vi "Diff_Drive_System_Act_AutoTune.vi"(6 "FPGA_Time_Seconds":dbl, 9 "Right Speed":dbl, 10 "Left Speed":dbl, 11 "Diff_Drive_Device_Refs":T1 {"GyroDevRef"."Sample Rate" min=0.25 max=100.0 step=0.25}) -> ()   [LabVIEW 2019]
uses:
  Diff_Drive_System_Device_Refs.ctl
  <vilib>/Rock Robotics/WPI/Gyro/WPI_GyroDevRef.ctl
  <vilib>/Rock Robotics/SystemInterfaces/AI/FPGA_AIChannel.ctl
  <vilib>/Rock Robotics/SystemInterfaces/spilib/spi_bus.ctl
  <vilib>/Rock Robotics/WPI/RobotDrive/WPI_RobotDriveDevRef.ctl
  <vilib>/Rock Robotics/WPI/MotorControl/WPI_MotorControlDeviceRef.ctl
  <vilib>/Rock Robotics/WPI/MotorControl/WPI_MotorControlType.ctl
  <vilib>/Rock Robotics/SystemInterfaces/DIO/FPGA_DIOPWMChannel.ctl
  <vilib>/Rock Robotics/WPI/PWM/WPI_PWMDeadband.ctl
  <vilib>/Rock Robotics/SystemInterfaces/DIO/FPGA_DIOChannel.ctl
  <vilib>/Rock Robotics/WPI/Encoder/WPI_EncoderDevRef.ctl
  <vilib>/Rock Robotics/SystemInterfaces/Encoder/FPGA_EncoderIdx.ctl
  <vilib>/Rock Robotics/SystemInterfaces/Counter/FPGA_CounterCtrSystemIndex.ctl
  <vilib>/Rock Robotics/WPI/Encoder/WPI_EncoderType.ctl
  <vilib>/Rock Robotics/WPI/ThirdParty/JAS_Junk/TrajLib/SlewRateLimiter_New.vi
  <vilib>/Rock Robotics/WPI/ThirdParty/JAS_Junk/TrajLib/SlewRateLimiter_Reset.vi
  <vilib>/Rock Robotics/WPI/ThirdParty/JAS_Junk/TrajLib/SlewRateLimiter_Calculate.vi
  <vilib>/Rock Robotics/WPI/ThirdParty/JAS_Junk/TrajLib/SlewRateLimiter_SetRate.vi
  <vilib>/Rock Robotics/WPI/ThirdParty/JAS_Junk/TrajLib/SimpleMotorFF_Calculate.vi
  <vilib>/Rock Robotics/WPI/ThirdParty/JAS_Junk/TrajLib/PIDController_AtSetpoint.vi
  <vilib>/Rock Robotics/WPI/ThirdParty/JAS_Junk/TrajLib/PIDController_SetPIDF.vi
  <vilib>/Rock Robotics/WPI/ThirdParty/JAS_Junk/TrajLib/PIDController_SetDerivativeFilter.vi
  <vilib>/Rock Robotics/WPI/ThirdParty/JAS_Junk/TrajLib/PIDController_SetIntegratorRange.vi
  <vilib>/Rock Robotics/WPI/ThirdParty/JAS_Junk/TrajLib/PIDController_SetTolerancePandV.vi
  <vilib>/Rock Robotics/WPI/ThirdParty/JAS_Junk/TrajLib/PIDController_DisableContinousInput.vi
  <vilib>/Rock Robotics/WPI/ThirdParty/JAS_Junk/TrajLib/PIDController_EnableContinousInput.vi
  <vilib>/Rock Robotics/WPI/ThirdParty/JAS_Junk/TrajLib/PIDController_Reset.vi
  <vilib>/Rock Robotics/WPI/ThirdParty/JAS_Junk/TrajLib/PIDController_New.vi
  <vilib>/Rock Robotics/WPI/ThirdParty/JAS_Junk/TrajLib/PIDController_SetOutputLimits.vi
  <vilib>/Rock Robotics/WPI/ThirdParty/JAS_Junk/TrajLib/PIDController_NewPeriod.vi
  <vilib>/Rock Robotics/SystemInterfaces/NetworkCommunication/NetComm_UsageReport_report.vi
  Diff_Drive_System_Globals.vi
  <vilib>/Rock Robotics/WPI/ThirdParty/JAS_Junk/TrajLib/Util_LibraryGlobals.vi
  <vilib>/Rock Robotics/WPI/ThirdParty/JAS_Junk/TrajLib/PIDController_AdvCalculate_FF_Sp_Pv.vi
  <vilib>/Rock Robotics/WPI/ThirdParty/JAS_Junk/TrajLib/Trajectory_Library.lvlib
panel:
  # "Analog"
  # "XRS"
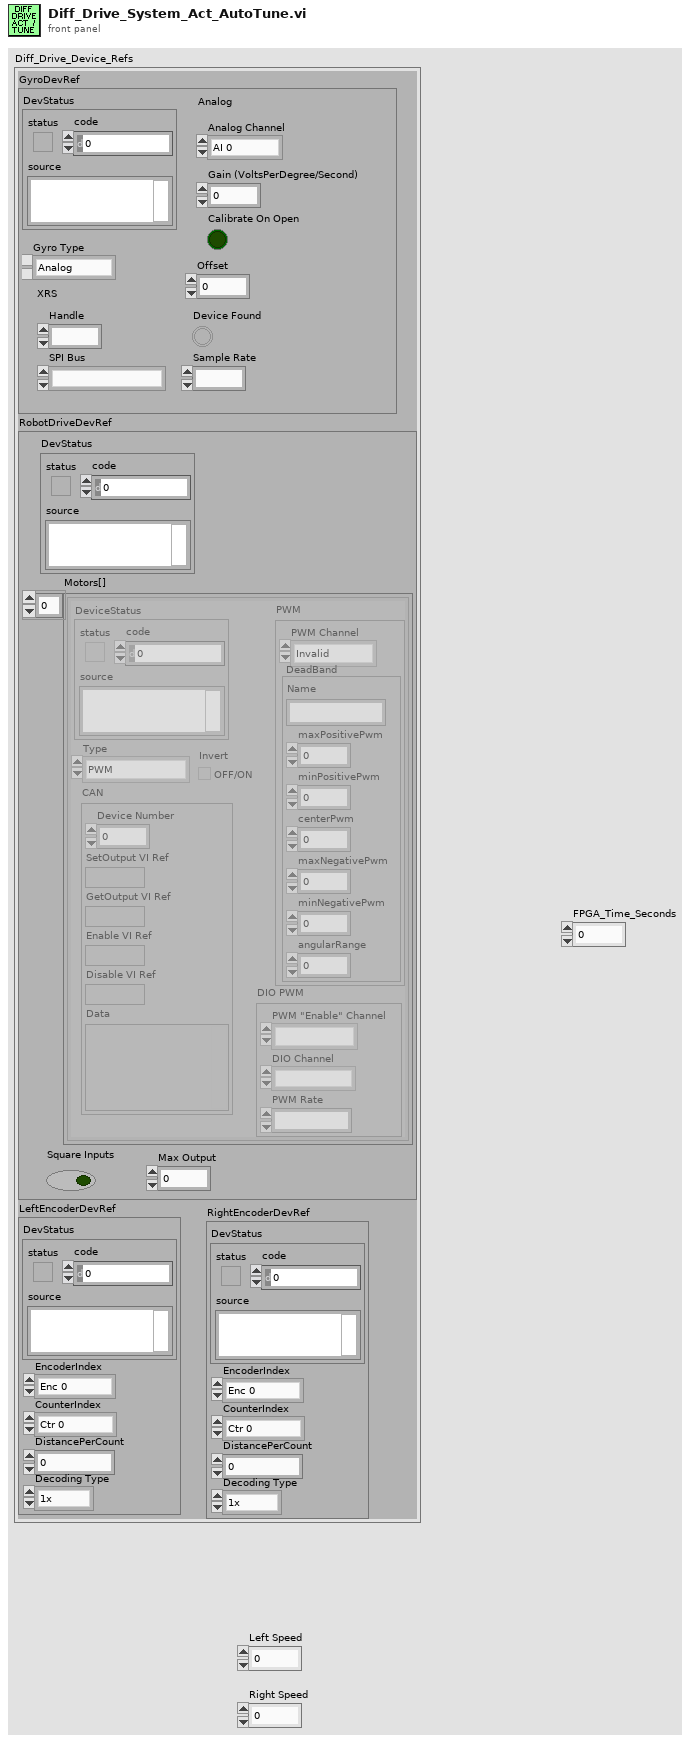
[diagram p1: front panel]
types:
  T1 = typedef "Diff_Drive_System_Device_Refs.ctl" = cluster{"GyroDevRef":T2, "RobotDriveDevRef":T5, "LeftEncoderDevRef":T11, "RightEncoderDevRef":T11}
  T2 = typedef "WPI_GyroDevRef.ctl" = cluster{"DevStatus":errorcluster, "Analog Channel":T3, "Gain (VoltsPerDegree/Second)":dbl, "Gyro Type":enum16{"Analog", "XRS450"}, "Handle":i32, "SPI Bus":T4, "Device Found":bool, "Sample Rate":dbl, "Calibrate On Open":bool, "Offset":dbl}
  T3 = typedef "FPGA_AIChannel.ctl" = enum8{"AI 0", "AI 1", "AI 2", "AI 3", "AI MXP 0", "AI MXP 1", "AI MXP 2", "AI MXP 3", "Invalid"}
  T4 = typedef "spi_bus.ctl" = enum16{"SPI On-Board, CS0", "SPI On-Board, CS1", "SPI On-Board, CS2", "SPI On-Board, CS3", "SPI MXP", "Invalid"}
  T5 = typedef "WPI_RobotDriveDevRef.ctl" = cluster{"DevStatus":errorcluster, "Motors[]":T6[], "Square Inputs":bool, "Max Output":dbl}
  T6 = typedef "WPI_MotorControlDeviceRef.ctl" = cluster{"DeviceStatus":errorcluster, "Type":T7, "PWM":cluster{"PWM Channel":T8, "DeadBand":T9}, "CAN":cluster{"Device Number":u8, "SetOutput VI Ref":variant, "GetOutput VI Ref":variant, "Enable VI Ref":variant, "Disable VI Ref":variant, "Data":variant}, "Invert":bool, "DIO PWM":cluster{"PWM \"Enable\" Channel":T8, "DIOChannel":T10, "PWM Rate":dbl}}
  T7 = typedef "WPI_MotorControlType.ctl" = enum16{"PWM", "CAN", "DIO PWM"}
  T8 = typedef "FPGA_DIOPWMChannel.ctl" = enum8{"PWM 0", "PWM 1", "PWM 2", "PWM 3", "PWM 4", "PWM 5", "PWM 6", "PWM 7", "PWM 8", "PWM 9", "PWM MXP 0", "PWM MXP 1", "PWM MXP 2", "PWM MXP 3", "PWM MXP 4", "PWM MXP 5", "PWM MXP 6", "PWM MXP 7", "PWM MXP 8", "PWM MXP 9", "Invalid"}
  T9 = typedef "WPI_PWMDeadband.ctl" = cluster{"Name":string, "maxPositivePwm":i32, "minPositivePwm":i32, "centerPwm":i32, "maxNegativePwm":i32, "minNegativePwm":i32, "angularRange":u16}
  T10 = typedef "FPGA_DIOChannel.ctl" = enum8{"DIO 0", "DIO 1", "DIO 2", "DIO 3", "DIO 4", "DIO 5", "DIO 6", "DIO 7", "DIO 8", "DIO 9", "DIO MXP 0", "DIO MXP 1", "DIO MXP 2", "DIO MXP 3", "DIO MXP 4", "DIO MXP 5", "DIO MXP 6", "DIO MXP 7", "DIO MXP 8", "DIO MXP 9", "DIO MXP 10", "DIO MXP 11", "DIO MXP 12", "DIO MXP 13", "DIO MXP 14", "DIO MXP 15", "SPI Port CS1", "SPI Port CS2", "SPI Port CS3", "SPI Port MISO", "SPI Port MOSI", "Invalid"}
  T11 = typedef "WPI_EncoderDevRef.ctl" = cluster{"DevStatus":errorcluster, "EncoderIndex":T12, "CounterIndex":T13, "DistancePerCount":dbl, "Decoding Type":T14}
  T12 = typedef "FPGA_EncoderIdx.ctl" = enum8{"Enc 0", "Enc 1", "Enc 2", "Enc 3", "Enc 4", "Enc 5", "Enc 6", "Enc 7", "Invalid"}
  T13 = typedef "FPGA_CounterCtrSystemIndex.ctl" = enum8{"Ctr 0", "Ctr 1", "Ctr 2", "Ctr 3", "Ctr 4", "Ctr 5", "Ctr 6", "Ctr 7", "Invalid"}
  T14 = typedef "WPI_EncoderType.ctl" = enum16{"1x", "2x", "4x"}
  T15 = enum16{"Ziegler Nicols - Fast", "Ziegler Nicols - Normal", "Ziegler Nicols - Slow", "CHR regulator - 0% overshoot", "CHR regulator - 20% overshoot", "CHR servo - 0 % overshoot", "CHR servo - 20% overshoot"}
  T16 = typedef "Trajectory_Library.lvlib/SIMPLE_MOTOR_FF.ctl" = cluster{"Ks":dbl, "Kv":dbl, "Ka":dbl, "KnInv":dbl}
  T17 = typedef "Trajectory_Library.lvlib/PID_ADV_LIMITS.ctl" = cluster{"MaxInput":dbl, "MinInput":dbl, "Continuous":bool, "MaxOutput":dbl, "MinOutput":dbl}
  T18 = typedef "Trajectory_Library.lvlib/PID_ADV_TUNING.ctl" = cluster{"Kf":dbl, "Kp":dbl, "Ki":dbl, "Kd":dbl, "MaximumIntegral":dbl, "MinimumIntegral":dbl, "Filter Derivative":bool}
  T19 = cluster{"Controller Constant Type":enum16{"Ziegler Nicols - Fast", "Ziegler Nicols - Normal", "Ziegler Nicols - Slow", "CHR regulator - 0% overshoot", "CHR regulator - 20% overshoot", "CHR servo - 0 % overshoot", "CHR servo - 20% overshoot"}, "Type of Controller":enum16{"P", "PI", "PID"}, "CO Offset":dbl, "Kn":dbl, "Tuning Tolerance":dbl, "Plant Tolerance":dbl, "Newest Avg Time ":i32, "Long Ave Time":i32}
  T20 = cluster{"proportional gain (Kp)":dbl, "integral time (Ki / Sec)":dbl, "derivative time (Kd /Sec)":dbl}
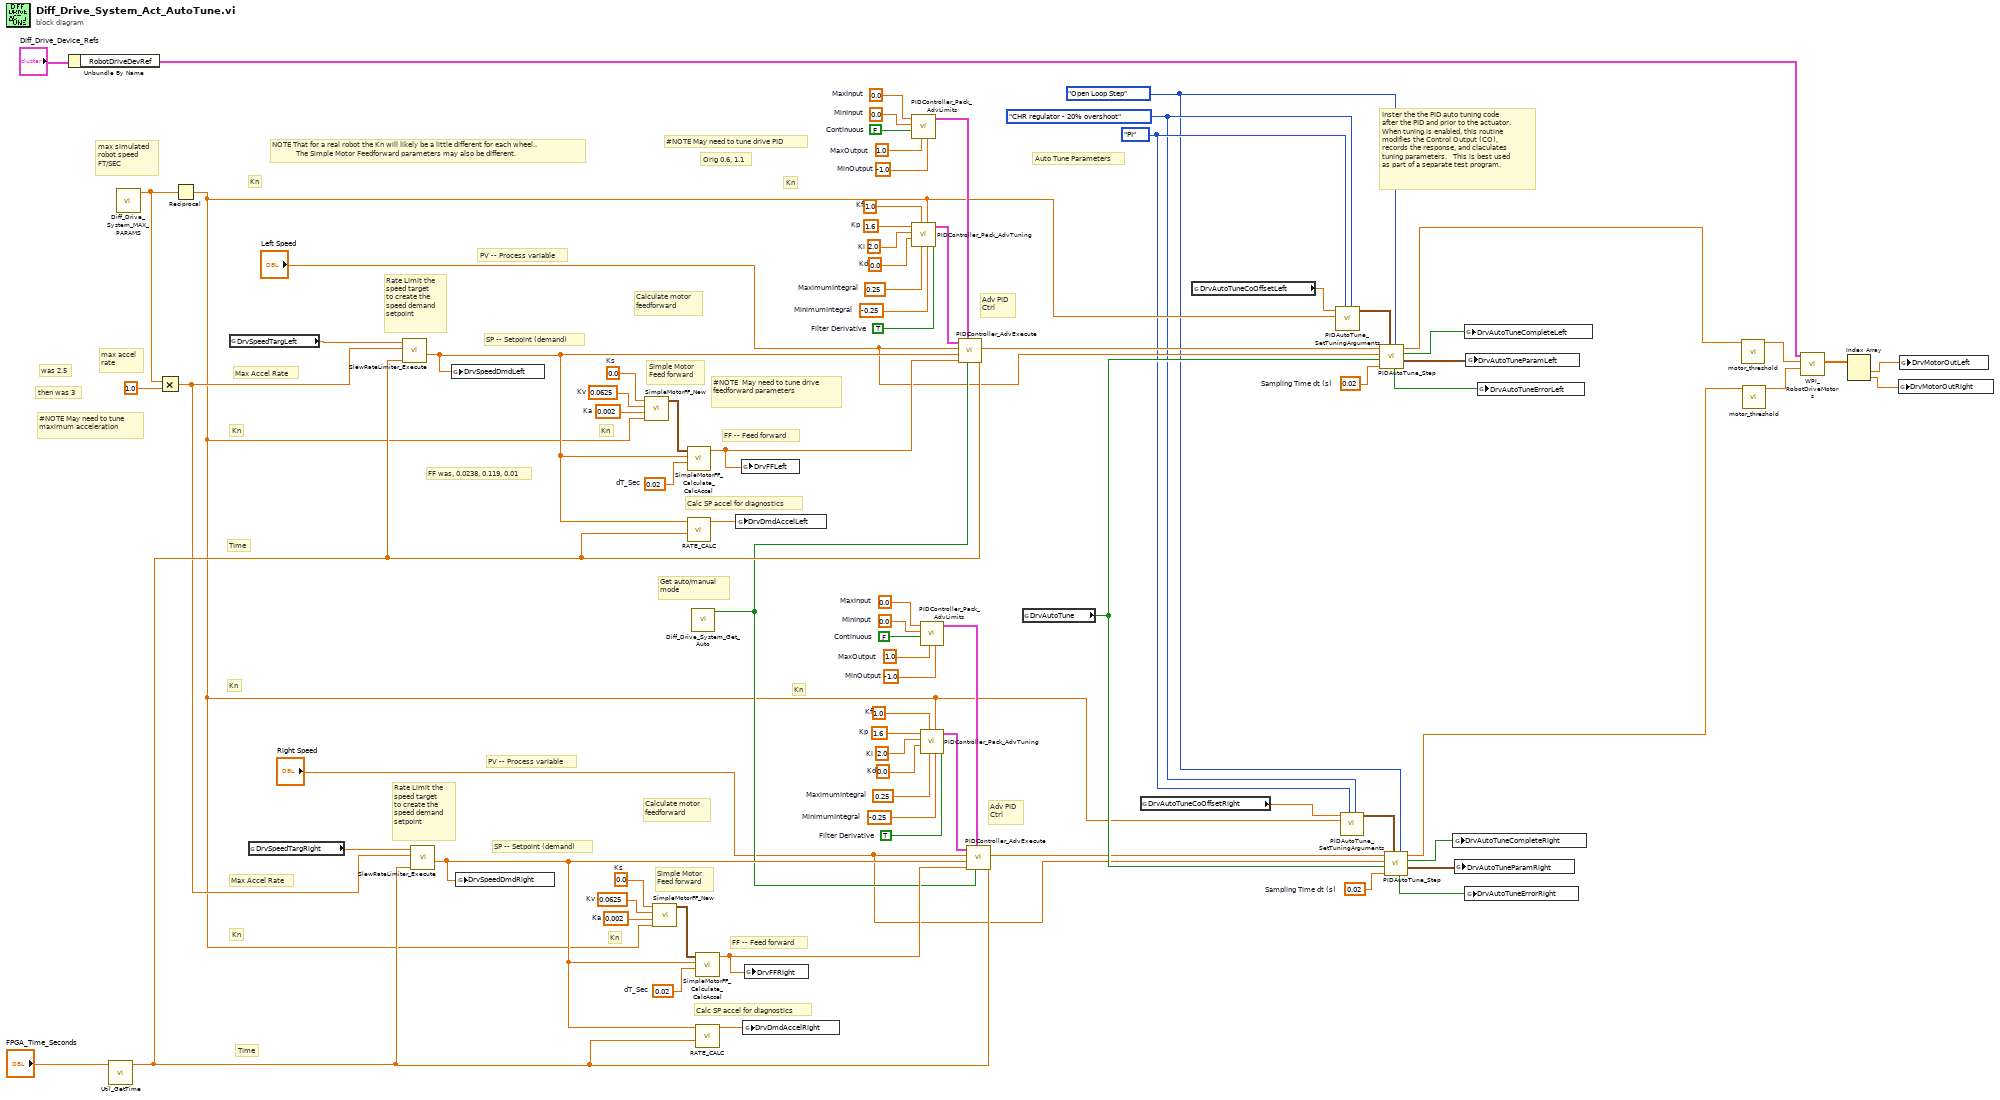
[diagram p0: block diagram]
diagram:
  w19 = 0.02  # Sampling Time dt (s)
  w1 = enum16{"Open Loop Step", "Closed Loop Step"}."Open Loop Step" ("Procedure Type")
  w2 = T15."CHR regulator - 20% overshoot" ("Controller Constant Type")
  w3 = enum16{"P", "PI", "PID"}."PI" ("Type of Controller")
  w24 = 0.02  # Sampling Time dt (s)
  w45 = 1.6  # Kp
  w44 = 2.0  # Ki
  w43 = 0.0  # Kd
  w42 = 1.0  # Kf
  w41 = 0.25  # MaximumIntegral
  w40 = -0.25  # MinimumIntegral
  w39 = TRUE  # Filter Derivative
  w37 = 0.0  # MinInput
  w36 = FALSE  # Continuous
  w35 = 1.0  # MaxOutput
  w38 = -1.0  # MinOutput
  w34 = 0.0  # MaxInput
  w50 = 0.02  # dT_Sec
  w48 = 0.0  # Ks
  w47 = 0.0625  # Kv
  w46 = 0.002  # Ka
  w68 = 1.6  # Kp
  w67 = 2.0  # Ki
  w66 = 0.0  # Kd
  w65 = 1.0  # Kf
  w64 = 0.25  # MaximumIntegral
  w63 = -0.25  # MinimumIntegral
  w62 = TRUE  # Filter Derivative
  w60 = 0.0  # MinInput
  w59 = FALSE  # Continuous
  w58 = 1.0  # MaxOutput
  w61 = -1.0  # MinOutput
  w57 = 0.0  # MaxInput
  w74 = 0.02  # dT_Sec
  w72 = 0.0  # Ks
  w71 = 0.0625  # Kv
  w70 = 0.002  # Ka
  # "Auto Tune Parameters"
  # "Inster the the PID auto tuning code\nafter the PID and prior to the actuator.\nWhen tuning is enabled, this routine\nmodifies the Control Output (CO), \nrecords the response, and claculates\ntuning parameters.   This is best used\nas part of a separate test program."
  # "Get auto/manual\nmode"
  # "then was 3"
  # "FF was, 0.0238, 0.119, 0.01"
  # "Orig 0.6, 1.1"
  # "NOTE That for a real robot the Kn will likely be a little different for each wheel..\n            The Simple Motor Feedforward parameters may also be different."
  # "Max Accel Rate"
  # "Max Accel Rate"
  # "Time"
  # "Kn"
  # "Kn"
  # "Kn"
  # "Kn"
  # "Time"
  # "Kn"
  # "PV -- Process variable"
  # "Kn"
  # "Calc SP accel for diagnostics"
  # "FF -- Feed forward"
  # "SP -- Setpoint (demand)"
  # "Adv PID\nCtrl"
  # "Calculate motor\nfeedforward"
  # "Rate Limit the \nspeed target\nto create the\nspeed demand\nsetpoint"
  # "Simple Motor\nFeed forward"
  # "Kn"
  # "PV -- Process variable"
  # "Kn"
  # "Calc SP accel for diagnostics"
  # "FF -- Feed forward"
  # "SP -- Setpoint (demand)"
  # "Adv PID\nCtrl"
  # "Calculate motor\nfeedforward"
  # "was 2.5"
  # "Rate Limit the \nspeed target\nto create the\nspeed demand\nsetpoint"
  # "Simple Motor\nFeed forward"
  # "#NOTE May need to tune drive PID"
  # "#NOTE May need to tune maximum acceleration"
  # "#NOTE  May need to tune drive feedforward parameters"
  # "max simulated\nrobot speed\nFT/SEC"
  # "max accel\nrate"
  n1 = Unbundle By Name("Diff_Drive_Device_Refs") -> ("RobotDriveDevRef"=w77:T5)
  n2 = call <vilib>:"Util_GetTime.vi"("Pass_Through_Time"="FPGA_Time_Seconds") -> ("FPGA_Time_Seconds"=w31:dbl)  [unwired: 9 in, 1 out]
  n3 = call "Diff_Drive_System_MAX_PARAMS.vi"() -> ("Max Speed Ft/Sec"=w52:dbl)  [unwired: 9 in, 2 out]
  n4 = Multiply(x=w52, y=1.0 ("x")) -> (x*y=w30:dbl)
  n5 = Reciprocal(x=w52) -> (1/x=w12:dbl)
  n6 = global read "Diff_Drive_System_Globals.vi" "DrvSpeedTargLeft"() -> (w69:dbl)
  n7 = global read "Diff_Drive_System_Globals.vi" "DrvSpeedTargRight"() -> (w29:dbl)
  n8 = call <vilib>:"SlewRateLimiter_Execute.vi"("Time"=w31, "PositiveRate"=w30, "Input"=w69) -> ("Output"=w54:dbl)  [unwired: 7 in, 1 out]
  n9 = call <vilib>:"SlewRateLimiter_Execute.vi"("Time"=w31, "PositiveRate"=w30, "Input"=w29) -> ("Output"=w26:dbl)  [unwired: 7 in, 1 out]
  n10 = global write "Diff_Drive_System_Globals.vi" "DrvSpeedDmdLeft"(w54) -> ()
  n11 = global write "Diff_Drive_System_Globals.vi" "DrvSpeedDmdRight"(w26) -> ()
  n12 = call <vilib>:"SimpleMotorFF_New.vi"("Kn"=w12, "Ka"=w70, "Kv"=w71, "Ks"=w72) -> ("SIMPLE_MOTOR_FF"=w73:T16)  [unwired: 7 in]
  n13 = call <vilib>:"SimpleMotorFF_New.vi"("Kn"=w12, "Ka"=w46, "Kv"=w47, "Ks"=w48) -> ("SIMPLE_MOTOR_FF"=w49:T16)  [unwired: 7 in]
  n14 = call <vilib>:"SimpleMotorFF_Calculate_CalcAccel.vi"("dT_Sec"=w74, "VelSp"=w54, "SIMPLE_MOTOR_FF"=w73) -> ("FeedForward"=w51:dbl)  [unwired: 8 in]
  n15 = call "RATE_CALC.vi"("Time"=w31, "Input"=w54) -> ("Output"=w53:dbl)  [unwired: 9 in]
  n16 = call "Diff_Drive_System_Get_Auto.vi"() -> ("Auto Mode"=w25:bool)  [unwired: 11 in]
  n17 = call <vilib>:"SimpleMotorFF_Calculate_CalcAccel.vi"("dT_Sec"=w50, "VelSp"=w26, "SIMPLE_MOTOR_FF"=w49) -> ("FeedForward"=w28:dbl)  [unwired: 8 in]
  n18 = call "RATE_CALC.vi"("Time"=w31, "Input"=w26) -> ("Output"=w27:dbl)  [unwired: 9 in]
  n19 = global write "Diff_Drive_System_Globals.vi" "DrvDmdAccelLeft"(w53) -> ()
  n20 = global write "Diff_Drive_System_Globals.vi" "DrvFFLeft"(w51) -> ()
  n21 = global write "Diff_Drive_System_Globals.vi" "DrvDmdAccelRight"(w27) -> ()
  n22 = global write "Diff_Drive_System_Globals.vi" "DrvFFRight"(w28) -> ()
  n23 = call <vilib>:"PIDController_Pack_AdvLimits.vi"("MinOutput"=w61, "MaxOutput"=w58, "Continuous"=w59, "MinInput"=w60, "MaxInput"=w57) -> ("Adv PID Limits"=w55:T17)  [unwired: 6 in]
  n24 = call <vilib>:"PIDController_Pack_AdvTuning.vi"("Filter Derivative"=w62, "MinimumIntegral"=w63, "Kn"=w12, "MaximumIntegral"=w64, "Kf"=w65, "Kd"=w66, "Ki"=w67, "Kp"=w68) -> ("Adv PID Tuning"=w56:T18)  [unwired: 3 in]
  n25 = call <vilib>:"PIDController_Pack_AdvLimits.vi"("MinOutput"=w38, "MaxOutput"=w35, "Continuous"=w36, "MinInput"=w37, "MaxInput"=w34) -> ("Adv PID Limits"=w32:T17)  [unwired: 6 in]
  n26 = call <vilib>:"PIDController_Pack_AdvTuning.vi"("Filter Derivative"=w39, "MinimumIntegral"=w40, "Kn"=w12, "MaximumIntegral"=w41, "Kf"=w42, "Kd"=w43, "Ki"=w44, "Kp"=w45) -> ("Adv PID Tuning"=w33:T18)  [unwired: 3 in]
  n27 = call <vilib>:"PIDController_AdvExecute.vi"("Time"=w31, "Auto"=w25, "Adv PID Limits"=w55, "FF-FeedForward"=w51, "SP-SetPoint"=w54, "PV-Measurement"="Left Speed", "Adv PID Tuning"=w56) -> ("CO-ControlOutput"=w21:dbl)  [unwired: 2 in, 2 out]
  n28 = call <vilib>:"PIDController_AdvExecute.vi"("Time"=w31, "Auto"=w25, "Adv PID Limits"=w32, "FF-FeedForward"=w28, "SP-SetPoint"=w26, "PV-Measurement"="Right Speed", "Adv PID Tuning"=w33) -> ("CO-ControlOutput"=w16:dbl)  [unwired: 2 in, 2 out]
  n29 = global read "Diff_Drive_System_Globals.vi" "DrvAutoTune"() -> (w17:bool)
  n30 = global read "Diff_Drive_System_Globals.vi" "DrvAutoTuneCoOffsetRight"() -> (w13:dbl)
  n31 = global read "Diff_Drive_System_Globals.vi" "DrvAutoTuneCoOffsetLeft"() -> (w14:dbl)
  n32 = call <vilib>:"PIDAutoTune_SetTuningArguments.vi"("Controller Constant Type"=w2, "Type of Controller"=w3, "Kn"=w12, "CO Offset"=w14) -> ("Configuration Parameters"=w23:T19)  [unwired: 7 in]
  n33 = call <vilib>:"PIDAutoTune_SetTuningArguments.vi"("Controller Constant Type"=w2, "Type of Controller"=w3, "Kn"=w12, "CO Offset"=w13) -> ("Configuration Parameters"=w18:T19)  [unwired: 7 in]
  n34 = call <vilib>:"PIDAutoTune_Step.vi"("Procedure Type"=w1, "Configuration Parameters"=w23, "Sampling Time dt (s)"=w24, "Tune"=w17, "Measurement  (PV)"="Left Speed", "Control Output (Co)"=w21) -> ("New Tuning Parameters"=w10:T20, "Tuning Done"=w11:bool, "Adj CO"=w20:dbl, "Error Occured"=w4:bool)  [unwired: 2 out]
  n35 = call <vilib>:"PIDAutoTune_Step.vi"("Procedure Type"=w1, "Configuration Parameters"=w18, "Sampling Time dt (s)"=w19, "Tune"=w17, "Measurement  (PV)"="Right Speed", "Control Output (Co)"=w16) -> ("New Tuning Parameters"=w8:T20, "Tuning Done"=w9:bool, "Adj CO"=w15:dbl, "Error Occured"=w5:bool)  [unwired: 2 out]
  n36 = global write "Diff_Drive_System_Globals.vi" "DrvAutoTuneCompleteRight"(w9) -> ()
  n37 = global write "Diff_Drive_System_Globals.vi" "DrvAutoTuneParamRight"(w8) -> ()
  n38 = global write "Diff_Drive_System_Globals.vi" "DrvAutoTuneCompleteLeft"(w11) -> ()
  n39 = global write "Diff_Drive_System_Globals.vi" "DrvAutoTuneErrorRight"(w5) -> ()
  n40 = global write "Diff_Drive_System_Globals.vi" "DrvAutoTuneParamLeft"(w10) -> ()
  n41 = global write "Diff_Drive_System_Globals.vi" "DrvAutoTuneErrorLeft"(w4) -> ()
  n42 = call "motor_threshold.vi"("motor in"=w20) -> ("motor out"=w22:dbl)  [unwired: 10 in]
  n43 = call "motor_threshold.vi"("motor in"=w15) -> ("motor out"=w81:dbl)  [unwired: 10 in]
  n44 = call <vilib>:"WPI_RobotDriveMotors.vi"("RightSpeed"=w81, "LeftSpeed"=w22, "RobotDriveDevRef"=w77) -> ("Motor Values"=w80:dbl[])  [unwired: 6 in, 2 out]
  n45 = Index Array(array=w80) -> (element #1=w76:dbl, element #2=w75:dbl)  [unwired: 2 in]
  n46 = global write "Diff_Drive_System_Globals.vi" "DrvMotorOutRight"(w75) -> ()
  n47 = global write "Diff_Drive_System_Globals.vi" "DrvMotorOutLeft"(w76) -> ()
